vi "AutoHelperSequencer_Example.vi"() -> ()   [LabVIEW 2019]
uses:
  <vilib>/Rock Robotics/WPI/ThirdParty/JAS_Junk/TrajLib/TypeDef/CHASSIS_SPEEDS.ctl
  <vilib>/Rock Robotics/WPI/ThirdParty/JAS_Junk/TrajLib/Enum/AutoHelperSequence_Step_Enum.ctl
  <vilib>/Rock Robotics/WPI/ThirdParty/JAS_Junk/TrajLib/VI/Util_GetTime_U32.vi
  <vilib>/Rock Robotics/WPI/ThirdParty/JAS_Junk/TrajLib/VI/DigSeqLogic_Edge_On.vi
  <vilib>/Rock Robotics/WPI/ThirdParty/JAS_Junk/TrajLib/Timer_New.vi
  <vilib>/Rock Robotics/WPI/ThirdParty/JAS_Junk/TrajLib/VI/Util_GetTime_U64.vi
  <vilib>/Utility/semaphor.llb/Obtain Semaphore Reference.vi
  <vilib>/Rock Robotics/WPI/ThirdParty/JAS_Junk/TrajLib/Timer_Reset.vi
  <vilib>/Rock Robotics/WPI/ThirdParty/JAS_Junk/TrajLib/VI/Timer_Restart.vi
  <vilib>/Rock Robotics/WPI/ThirdParty/JAS_Junk/TrajLib/Timer_HasPeriodPassedOnce.vi
  <vilib>/Rock Robotics/WPI/ThirdParty/JAS_Junk/TrajLib/Trajectory_Library.lvlib
panel:
  out "Auto \nFinished":bool
  out "Elapsed Step Time":dbl
  out "Step Number State":T1
  out "Output 2":bool
  out "Output 1":bool
  out "CHASSIS\nSpeed\nDemand":T2 {"vOmega" format="%10.3f"; "vY" format="%10.3f"; "vX" format="%10.3f"}
  in  "Run Auto":bool
  out "Waveform Chart":cluster{i16, i16}(graph)
  # "AUTO HELPER SEQUENCER EXAMPLE"
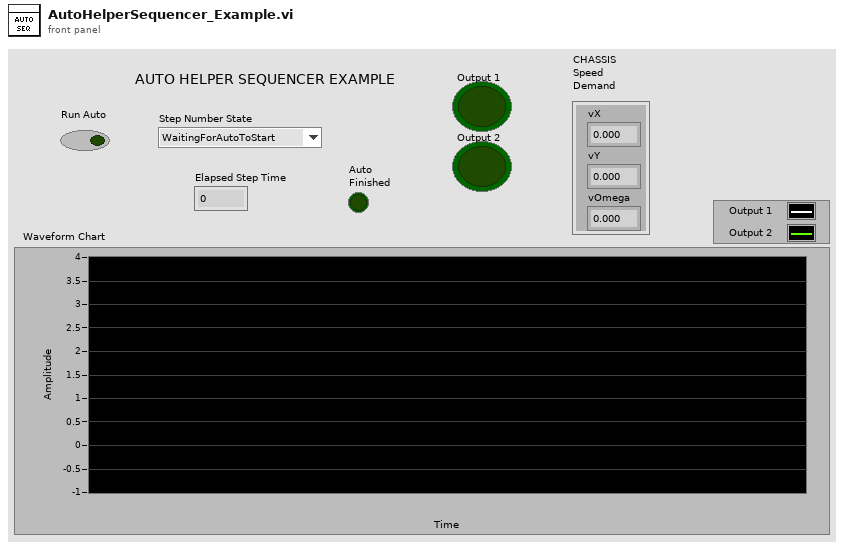
[diagram p1: front panel]
types:
  T1 = typedef "Trajectory_Library.lvlib/AutoHelperSequence_Step_Enum.ctl" = enum16{"WaitingForAutoToStart", "Step 1", "Step 2", "Step 3", "Step 4", "Step 5", "Step 6", "Step 7", "Step 8", "Step 9", "Step 10", "Step 11", "Step 12", "Step 13", "Step 14", "Step 15", "Step 16", "Step 17", "Step 18", "Step 19", "Step 20", "Step 21", "Step 22", "Step 23", "Step 24", "Step 25", "Step 26", "Step 27", "Step 28", "Step 29", "Step 30", "Step 31", "Step 32", "AutoDone"}
  T2 = typedef "Trajectory_Library.lvlib/CHASSIS_SPEEDS.ctl" = cluster{"vX":dbl, "vY":dbl, "vOmega":dbl}
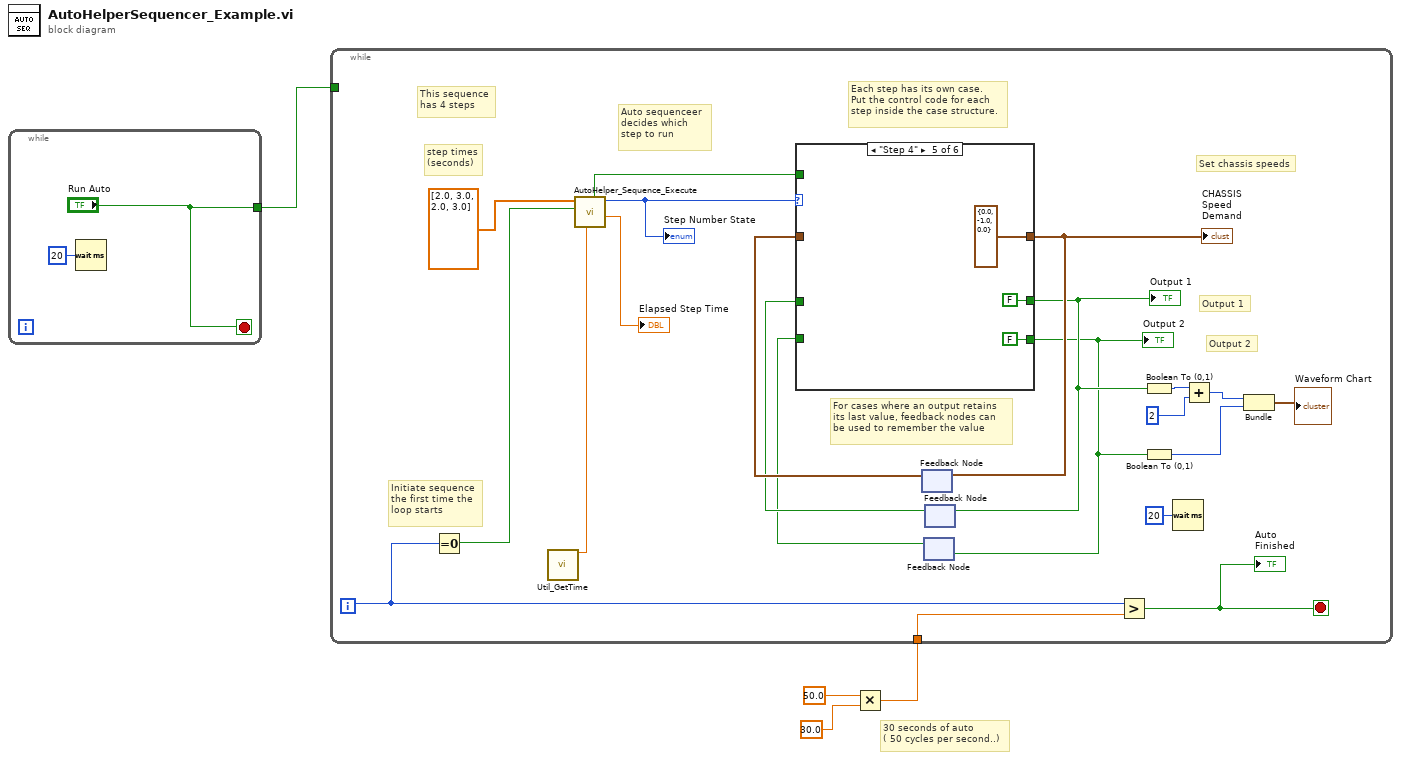
[diagram p0: block diagram]
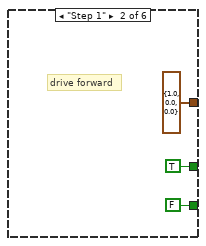
[diagram p3: hidden frame]
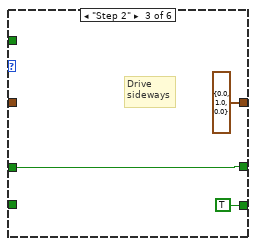
[diagram p4: hidden frame]
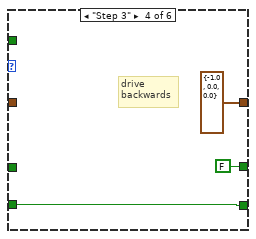
[diagram p5: hidden frame]
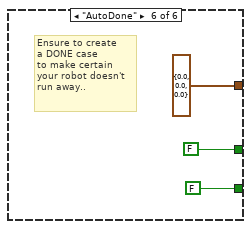
[diagram p6: hidden frame]
diagram:
  # "30 seconds of auto\n( 50 cycles per second..)"
  n1 = while {
    tunnel: ["Run Auto"] -> w4
    stop <- "Run Auto" stop-if-true
    n2 = Wait (ms)(milliseconds to wait=u32 20) -> ()  [unwired: 1 out]
  }
  n3 = Multiply(x=50.0, y=30.0) -> (x*y=w1:dbl)
  n4 = while {
    tunnel: w4 -> [_]
    tunnel: w1 -> [w8]
    i -> [w9]
    stop <- w7 stop-if-true
    # "step times\n(seconds)"
    # "This sequence\nhas 4 steps"
    # "Set chassis speeds"
    # "For cases where an output retains\nits last value, feedback nodes can \nbe used to remember the value"
    # "Output 2"
    # "Output 1"
    # "Each step has its own case.\nPut the control code for each\nstep inside the case structure."
    # "Auto sequenceer\ndecides which\nstep to run"
    # "Initiate sequence\nthe first time the \nloop starts"
    n5 = Equal To 0?(x=w9) -> (x = 0?=w20:bool)
    n6 = call <vilib>:"Util_GetTime.vi"() -> ("FPGA_Time_Seconds"=w19:dbl)  [unwired: 9 in, 2 out]
    n7 = call <vilib>:"AutoHelper_Sequence_Execute.vi"("Pass_Through_Time"=w19, "Initiate"=w20, "Step Times Sec"=dbl[] [2.0, 3.0, 2.0, 3.0]) -> ("Elapsed Step Time"=→"Elapsed Step Time":dbl, "Step Number State"=w18:T1, "New Step"=w11:bool)  [unwired: 4 in, 2 out]
    "Step Number State" <- w18
    n8 = feedback #1() -> (w16:T2)  [unwired: 1 in]
    n9 = feedback #2() -> (w14:bool)  [unwired: 1 in]
    n10 = feedback #3() -> (w15:bool)  [unwired: 1 in]
    n11 = case shown="\"Step 4\"" w18 {
      tunnel: [w29 TRUE w36 FALSE FALSE FALSE] -> w13
      tunnel: [w30 T2 {"vX"=1.0, "vY"=0.0, "vOmega"=0.0} T2 {"vX"=0.0, "vY"=1.0, "vOmega"=0.0} T2 {"vX"=-1.0, "vY"=0.0, "vOmega"=0.0} T2 {"vX"=0.0, "vY"=-1.0, "vOmega"=0.0} T2 {"vX"=0.0, "vY"=0.0, "vOmega"=0.0}] -> w17
      tunnel: [w28 FALSE TRUE w38 FALSE FALSE] -> w12
      tunnel: w16 -> [w30 _ _ _ _ _]
      tunnel: w15 -> [w29 _ w36 _ _ _]
      tunnel: w14 -> [w28 _ _ w38 _ _]
      tunnel: w11 -> [_ _ _ _ _ _]
      frame "WaitingForAutoToStart", Default {
      }
      frame "Step 1" {
        # "drive forward"
      }
      frame "Step 2" {
        # "Drive \nsideways"
      }
      frame "Step 3" {
        # "drive\nbackwards"
      }
      frame "Step 4" {
      }
      frame "AutoDone" {
        # "Ensure to create\na DONE case\nto make certain\nyour robot doesn't\nrun away.."
      }
    }
    "CHASSIS\nSpeed\nDemand" <- w17
    "Output 1" <- w13
    "Output 2" <- w12
    n12 = feedback-in #1(w17) -> ()
    n13 = feedback-in #2(w12) -> ()
    n14 = feedback-in #3(w13) -> ()
    n15 = Greater?(x=w9, y=w8) -> (0:w7:bool)
    "Auto \nFinished" <- w7
    n16 = Boolean To (0,1)(Boolean=w13) -> (0, 1=w24:i16)
    n17 = Boolean To (0,1)(Boolean=w12) -> (0, 1=w22:i16)
    n18 = Wait (ms)(milliseconds to wait=u32 20) -> ()  [unwired: 1 out]
    n19 = Add(x=w24, y=i16 2) -> (x+y=w23:i16)
    n20 = Bundle(w23, w22) -> (→"Waveform Chart":cluster{i16, i16})  [unwired: 1 in]
  }
